vi "translate_3d.vi"(6 "XYZ position":T1(array[cluster]), 9 "Point selection":enum16{"Light 0", "Light 1", "Ref point"}(ring), 10 "Zero":bool, 11 "Offset mode":enum32{"Absolute", "Relative"}(radio)) -> (1 "XYZ offsets":waveform(dbl)[](array[waveform]), 2 "Angles":cluster{"Altitude":dbl, "Azimuth":dbl} {"Azimuth" format="%7.3f"; "Altitude" format="%7.3g"}, 3 "Position":cluster{"X":dbl, "Y":dbl, "Z":dbl} {"Z" format="%#5.0g"; "Y" format="%#5.0g"; "X" format="%#5.0g"})   [LabVIEW 2010]
panel:
  in  "Relative offset":dbl[][](array[numeric])=[[-24.407620474133978, 95.2029577191849, -419.0563740301256], [-1326.037243034258, -4754.2110590937, -5183.668857122599], [-1904.8611007002526, -6910.705165242045, -7302.45249774368], [0.0, 0.0, -2.879363685972997]]
  # "(degrees)"
  # "(microns)"
  # "(mm)"
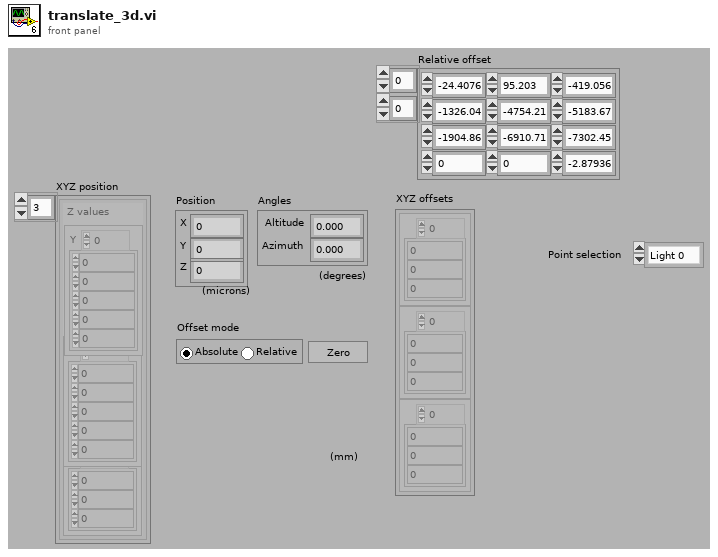
[diagram p1: front panel]
types:
  T1 = cluster{"Z values":waveform(dbl), "Y values":waveform(dbl), "Z values":waveform(dbl)}[]
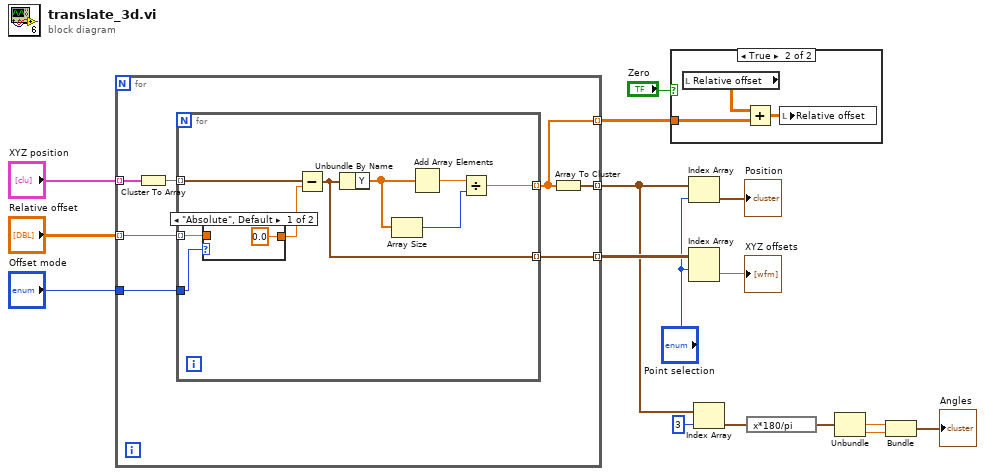
[diagram p0: block diagram]
diagram:
  n1 = for {
    tunnel: [w23] -> w7 mode=indexing
    tunnel: "XYZ position" -> [w21] mode=indexing
    tunnel: "Offset mode" -> [w20]
    tunnel: [w19] -> w12 mode=indexing
    tunnel: "Relative offset" -> [w17] mode=indexing
    tunnel: [w18] -> w9 mode=indexing
    n2 = Cluster To Array(cluster=w21) -> (array=w22:waveform(dbl)[])
    n3 = for {
      tunnel: w22 -> [w28] mode=indexing
      tunnel: [w29] -> w18 mode=indexing
      tunnel: w20 -> [w27]
      tunnel: [w25] -> w19 mode=indexing
      tunnel: w17 -> [w24] mode=indexing
      n4 = case shown="\"Absolute\", Default" w27 {
        tunnel: [0.0 ("[0]") w34] -> w26
        tunnel: w24 -> [_ w34]
        frame "Absolute", Default {
        }
        frame "Relative" {
        }
      }
      n5 = Subtract(x=w28, y=w26) -> (x-y=w25:waveform(dbl))
      n6 = Unbundle By Name(w25) -> ("Y"=w32:dbl[])
      n7 = Array Size(array=w32) -> (size(s)=w30:i32)
      n8 = Add Array Elements(numeric array=w32) -> (sum=w31:dbl)
      n9 = Divide(x=w31, y=w30) -> (x/y=w29:dbl)
    }
    n10 = Array To Cluster(array=w18) -> (cluster=w23:cluster{"[0]":dbl, "[1]":dbl, "[2]":dbl})
  }
  n11 = case shown="True" "Zero" {
    tunnel: w9 -> [_ w37]
    frame False {
    }
    frame True {
      n12 = local read "Relative offset"() -> (w36:dbl[][])
      n13 = Add(x=w36, y=w37) -> (x+y=w35:dbl[][])
      n14 = local write "Relative offset"(w35) -> ()
    }
  }
  n15 = Index Array(array=w7, index="Point selection") -> (element=→"Position":cluster{"[0]":dbl, "[1]":dbl, "[2]":dbl})
  n16 = Index Array(array=w12, index (row)="Point selection") -> (element=→"XYZ offsets":waveform(dbl)[])  [unwired: 1 in]
  n17 = Index Array(array=w7, index=3) -> (element=w5:cluster{"[0]":dbl, "[1]":dbl, "[2]":dbl})
  n18 = expression code="x*180/pi"(w5) -> (w4:cluster{"[0]":dbl, "[1]":dbl, "[2]":dbl})
  n19 = Unbundle(w4) -> ("[1]"=w3:dbl, "[2]"=w2:dbl)  [unwired: 1 out]
  n20 = Bundle("[1]"=w3, "[2]"=w2) -> (→"Angles":cluster{"[1]":dbl, "[2]":dbl})  [unwired: 1 out]
